vi "Exp no 4c Half Subtractor.vi"() -> ()   [LabVIEW 2010]
panel:
  out "BORROW":bool
  out "DIFFERENCE":bool
  in  "B":bool
  in  "A":bool
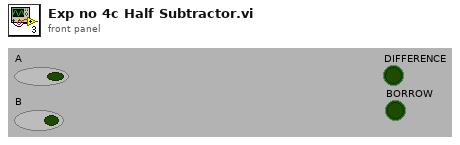
[diagram p1: front panel]
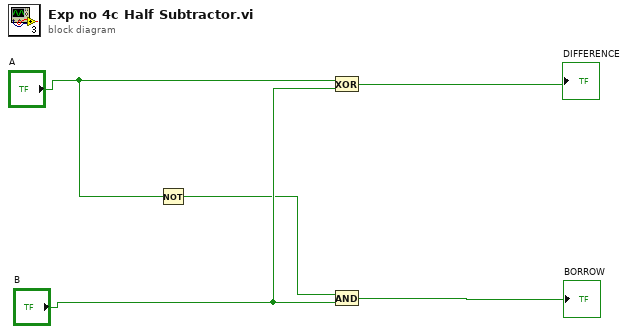
[diagram p0: block diagram]
diagram:
  n1 = Not(x="A") -> (.not. x?=w3:bool)
  n2 = Exclusive Or(1:"B", 2:"A") -> (0:→"DIFFERENCE":bool)
  n3 = And(x=w3, y="B") -> (x .and. y?=→"BORROW":bool)
